vi "Actual Record Length.vi"(8 "error in (no error)":errorcluster {"code" format="%.0x"}, 11 "VISA Resource Name":refnum<visa-resource-name>) -> (0 "error out":errorcluster {"code" format="%.0x"}, 1 "Actual Record Length":i32, 3 "VISA Resource Name Out":refnum<visa-resource-name>)   [LabVIEW 2010, in "Tektronix TDS 3000 Series.lvlib"]
doc: "This VI returns the actual number of points the oscilloscope acquires for each channel. After you configure the oscilloscope for an acquisition, call this VI to determine the size of the waveforms that the oscilloscope acquires. The value is equal to or greater than the minimum number of points you specify in the tktds3k Configure Acquisition Record VI. \n\nNotes:\n\n(1) The oscilloscope uses different size records depending on the acquisition type. You specify the acquisition type with the tktds3k Configure Acquisition Type VI."
uses:
  <instrlib>/Tektronix TDS 3000 Series/Tektronix TDS 3000 Series.lvlib
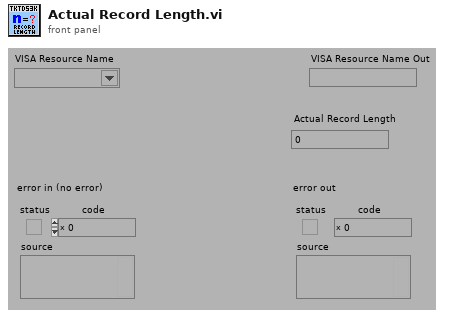
[diagram p1: front panel]
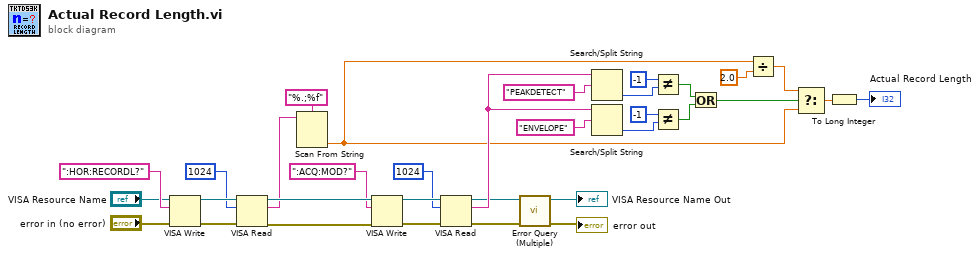
[diagram p0: block diagram]
diagram:
  n1 = VISA Write(VISA resource name="VISA Resource Name", write buffer=":HOR:RECORDL?", error in (no error)="error in (no error)") -> (VISA resource name out=w33:refnum<visa-resource-name>, error out=w30:errorcluster)  [unwired: 1 out]
  n2 = VISA Read(VISA resource name=w33, byte count=u32 1024 ("byte count (0)"), error in (no error)=w30) -> (VISA resource name out=w16:refnum<visa-resource-name>, read buffer=w7:string, error out=w15:errorcluster)  [unwired: 1 out]
  n3 = Scan From String(format string="%.;%f", input string=w7) -> (output 1=w5:dbl)  [unwired: 3 in, 3 out]
  n4 = VISA Write(VISA resource name=w16, write buffer=":ACQ:MOD?", error in (no error)=w15) -> (VISA resource name out=w26:refnum<visa-resource-name>, error out=w27:errorcluster)  [unwired: 1 out]
  n5 = VISA Read(VISA resource name=w26, byte count=u32 1024 ("byte count (0)"), error in (no error)=w27) -> (VISA resource name out=w2:refnum<visa-resource-name>, read buffer=w14:string, error out=w1:errorcluster)  [unwired: 1 out]
  n6 = call <instrlib>:"Error Query (Multiple).vi"("error in (no error)"=w1, "VISA Resource Name"=w2) -> ("error out"=→"error out":errorcluster, "VISA Resource Name Out"=→"VISA Resource Name Out":refnum<visa-resource-name>)  [unwired: 6 in, 2 out]
  n7 = Search/Split String(string=w14, search string/char (-)="PEAKDETECT") -> (offset of match=w23:i32)  [unwired: 1 in, 2 out]
  n8 = Search/Split String(string=w14, search string/char (-)="ENVELOPE") -> (offset of match=w20:i32)  [unwired: 1 in, 2 out]
  n9 = Not Equal?(x=-1, y=w23) -> (x != y?=w18:bool)
  n10 = Not Equal?(x=-1, y=w20) -> (x != y?=w17:bool)
  n11 = Or(x=w18, y=w17) -> (x .or. y?=w11:bool)
  n12 = Divide(x=w5, y=2.0) -> (x/y=w9:dbl)
  n13 = Select(t=w9, s=w11, f=w5) -> (s? t:f=w8:dbl)
  n14 = To Long Integer(number=w8) -> (32bit integer=→"Actual Record Length":i32)
